vi "Read from PGSQL.vi"(8 "error in (no error)":errorcluster, 10 "path":string, 11 "Logger in":refnum<class "Logger.PGSQL.lvclass">) -> (0 "error out":errorcluster, 1 "Variant":variant, 3 "Logger out":refnum<class "Logger.PGSQL.lvclass">)   [LabVIEW 2019, in "Logger.PGSQL.lvclass"]
uses:
  Logger.PGSQL.lvclass
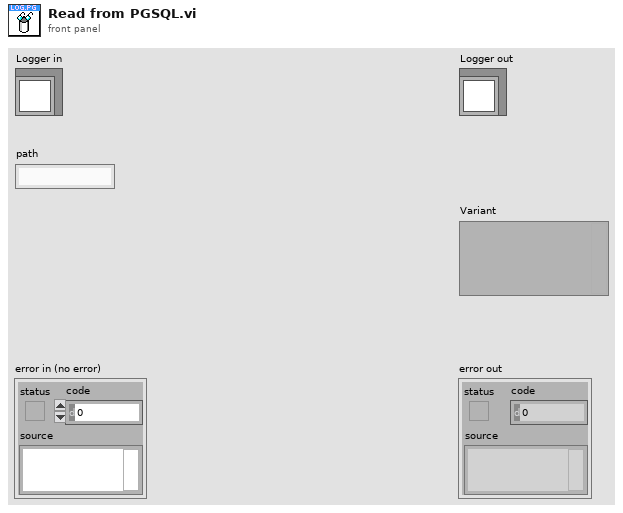
[diagram p1: front panel]
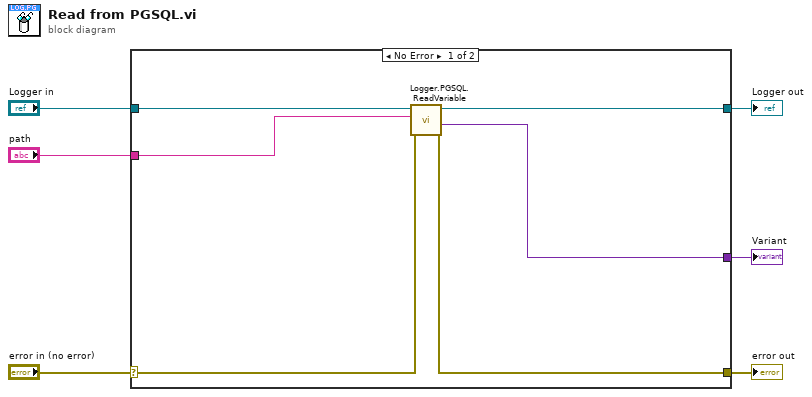
[diagram p0: block diagram]
diagram:
  n1 = case shown="No Error" "error in (no error)" {
    selector: "error in (no error)" -> [w10 w14]
    tunnel: [w9 w14] -> w5
    tunnel: [w12 w13] -> w3
    tunnel: "Logger in" -> [w8 w13]
    tunnel: "path" -> [w11 _]
    tunnel: [w7 _] -> w1
    frame No Error {
      n2 = call "Logger.PGSQL.ReadVariable.vi"("error in (no error)"=w10, "Address"=w11, "Logger"=w8) -> ("error out"=w9:errorcluster, "Data"=w7:variant, "Logger out"=w12:refnum<class "Logger.PGSQL.lvclass">)  [unwired: 6 in]
    }
    frame Error {
    }
  }
  "error out" <- w5
  "Logger out" <- w3
  "Variant" <- w1
